vi "XY_conf.vi"(3 "error in (no error)":errorcluster caption="错误输入（无错误）", 4 "方式":enum16{"写入", "读取"}(ring), 5 "XY图引用":refnum<vi>) -> (0 "error out":errorcluster caption="错误输出")   [LabVIEW 2020]
uses:
  <vilib>/Utility/config.llb/Read Key (Double).vi
  <vilib>/Utility/config.llb/Write Key (Double).vi
  <vilib>/Utility/config.llb/NI_LVConfig.lvlib
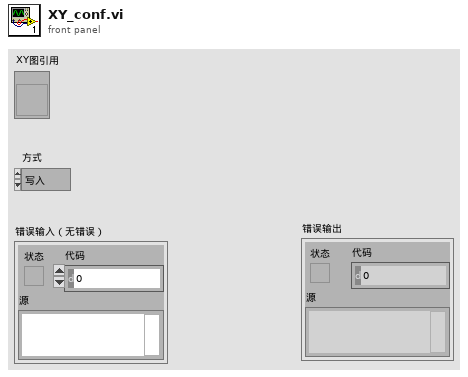
[diagram p1: front panel]
types:
  T1 = typedef "NI_LVConfig.lvlib/Config Data RefNum.ctl" = refnum<k1>
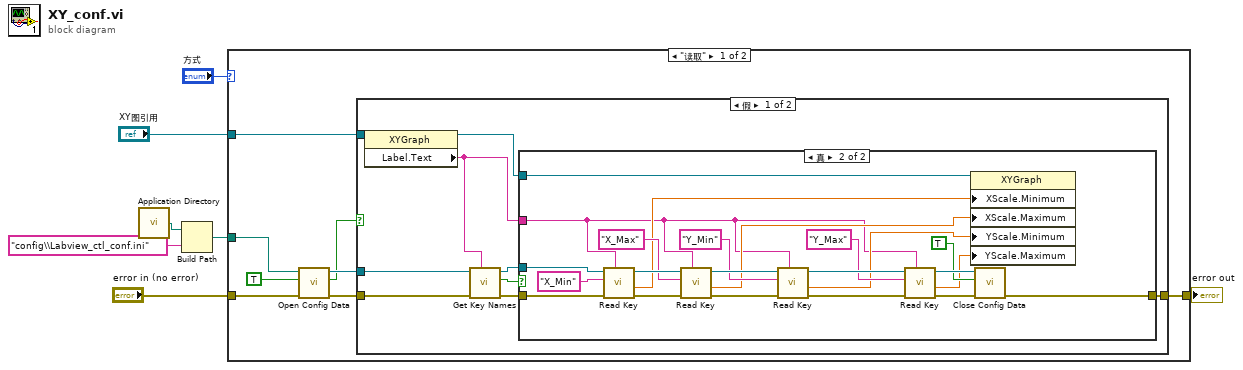
[diagram p0: block diagram]
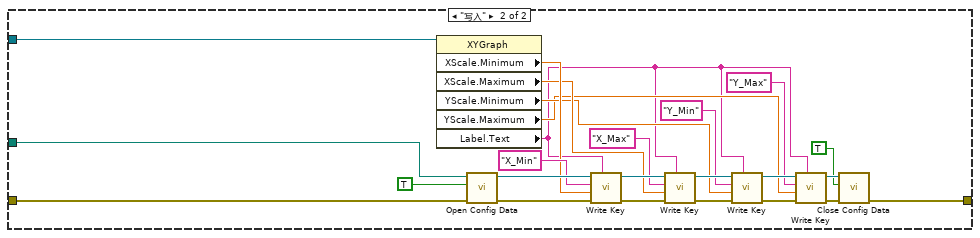
[diagram p4: hidden frame]
diagram:
  n1 = call <vilib>:"Application Directory.vi"() -> ("Application Directory"=w1:path)
  n2 = Build Path(base path=w1, name or relative path="config\\Labview_ctl_conf.ini" ("名称或相对路径")) -> (appended path=w4:path)
  n3 = case shown="\"读取\"" "方式" {
    tunnel: "XY图引用" -> [w11 w73]
    tunnel: w4 -> [w14 w71]
    tunnel: "error in (no error)" -> [w13 w68]
    tunnel: [w12 w54] -> w2
    frame "读取" {
      n4 = call <vilib>:"Open Config Data.vi"("error in (no error)"=w13, "create file if necessary (T)"=TRUE, "configuration file path"=w14) -> ("error out"=w9:errorcluster, "file created?"=w8:bool, "refnum"=w10:T1)  [unwired: 6 in]
      n5 = case shown="假" w8 {
        tunnel: [w24 w48] -> w12
        tunnel: w11 -> [w23 _]
        tunnel: w10 -> [w21 _]
        tunnel: w9 -> [w20 w48]
        frame False {
          n6 = property class="XYGraph"(reference=w23) -> (reference out=w22:refnum<vi>, "Label.Text"=w17:string)  [unwired: 1 in, 1 out]
          n7 = call <vilib>:"Get Key Names.vi"("section"=w17, "error in (no error)"=w20, "refnum"=w21) -> ("error out"=w19:errorcluster, "section exists?"=w16:bool, "refnum out"=w18:T1)  [unwired: 5 in, 1 out]
          n8 = case shown="真" w16 {
            tunnel: [w25 w35] -> w24
            tunnel: w22 -> [_ w33]
            tunnel: w19 -> [w25 w28]
            tunnel: w18 -> [_ w27]
            tunnel: w17 -> [_ w26]
            frame False {
            }
            frame True {
              n9 = call-poly <vilib>:"Read Key.vi"("section"=w26, "error in (no error)"=w28, "key"="X_Min", "refnum"=w27) -> ("error out"=w39:errorcluster, "value"=w32:dbl, "refnum out"=w46:T1)  [unwired: 4 in, 1 out]
              n10 = call-poly <vilib>:"Read Key.vi"("section"=w26, "error in (no error)"=w39, "key"="X_Max", "refnum"=w46) -> ("error out"=w38:errorcluster, "value"=w31:dbl, "refnum out"=w45:T1)  [unwired: 4 in, 1 out]
              n11 = call-poly <vilib>:"Read Key.vi"("section"=w26, "error in (no error)"=w38, "key"="Y_Min", "refnum"=w45) -> ("error out"=w37:errorcluster, "value"=w30:dbl, "refnum out"=w44:T1)  [unwired: 4 in, 1 out]
              n12 = call-poly <vilib>:"Read Key.vi"("section"=w26, "error in (no error)"=w37, "key"="Y_Max", "refnum"=w44) -> ("error out"=w36:errorcluster, "value"=w29:dbl, "refnum out"=w43:T1)  [unwired: 4 in, 1 out]
              n13 = property class="XYGraph"(reference=w33, "XScale.Minimum"=w32, "XScale.Maximum"=w31, "YScale.Minimum"=w30, "YScale.Maximum"=w29) -> ()  [unwired: 1 in, 2 out]
              n14 = call <vilib>:"Close Config Data.vi"("error in (no error)"=w36, "write file if changed (T)"=TRUE, "refnum"=w43) -> ("error out"=w35:errorcluster)  [unwired: 7 in, 1 out]
            }
          }
        }
        frame True {
        }
      }
    }
    frame "写入" {
      n15 = property class="XYGraph"(reference=w73) -> ("XScale.Minimum"=w66:dbl, "XScale.Maximum"=w53:dbl, "YScale.Minimum"=w52:dbl, "YScale.Maximum"=w51:dbl, "Label.Text"=w50:string)  [unwired: 1 in, 2 out]
      n16 = call <vilib>:"Open Config Data.vi"("error in (no error)"=w68, "create file if necessary (T)"=TRUE, "configuration file path"=w71) -> ("error out"=w69:errorcluster, "refnum"=w70:T1)  [unwired: 6 in, 1 out]
      n17 = call-poly <vilib>:"Write Key.vi"("section"=w50, "error in (no error)"=w69, "value"=w66, "key"="X_Min", "refnum"=w70) -> ("error out"=w58:errorcluster, "refnum out"=w65:T1)  [unwired: 4 in, 1 out]
      n18 = call-poly <vilib>:"Write Key.vi"("section"=w50, "error in (no error)"=w58, "value"=w53, "key"="X_Max", "refnum"=w65) -> ("error out"=w57:errorcluster, "refnum out"=w64:T1)  [unwired: 4 in, 1 out]
      n19 = call-poly <vilib>:"Write Key.vi"("section"=w50, "error in (no error)"=w57, "value"=w52, "key"="Y_Min", "refnum"=w64) -> ("error out"=w56:errorcluster, "refnum out"=w63:T1)  [unwired: 4 in, 1 out]
      n20 = call-poly <vilib>:"Write Key.vi"("section"=w50, "error in (no error)"=w56, "value"=w51, "key"="Y_Max", "refnum"=w63) -> ("error out"=w55:errorcluster, "refnum out"=w62:T1)  [unwired: 4 in, 1 out]
      n21 = call <vilib>:"Close Config Data.vi"("error in (no error)"=w55, "write file if changed (T)"=TRUE, "refnum"=w62) -> ("error out"=w54:errorcluster)  [unwired: 7 in, 1 out]
    }
  }
  "error out" <- w2
